vi "createInclinationFrame.vi"(8 "error in (no error)":errorcluster, 9 "TriggerIRQ":bool, 10 "WaitForTrigger":bool, 11 "MIILC in":refnum<class "MIILC.lvclass">) -> (0 "error out":errorcluster, 2 "TxFrame":T1 {"Data" format="%02x"}, 3 "MIILC out":refnum<class "MIILC.lvclass">)   [LabVIEW 2016, in "RTMIILC.lvlib" / "MIILC.lvclass"]
uses:
  MIILC.lvclass
  D:/Code/Common_RT_ILC/ILC/ILC.lvclass
  Common_RT_Modbus/DataTypes/TxFrame.ctl
  Common_RT_Modbus/DynamicFrameBuilder/DynamicFrameBuilder.lvclass
  MIILC.lvclass/MIILC.ctl
  Common_RT_ILC/ILC/ILC.lvclass/ILC.ctl
  Common_RT_ILC/ILC/ILC.lvclass
  Common_RT_Modbus/RTModbus.lvlib
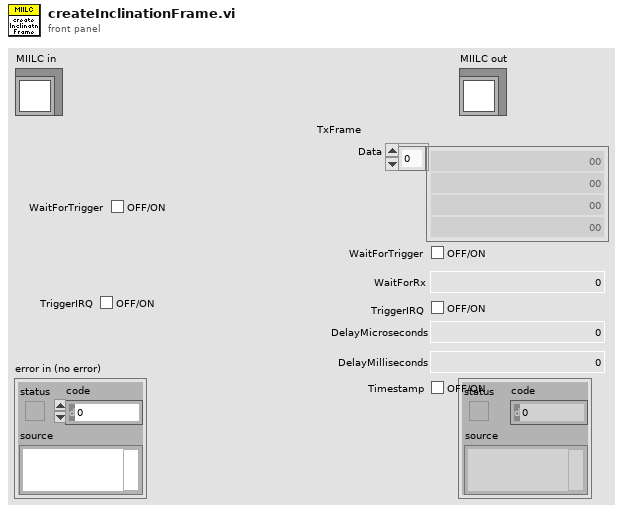
[diagram p1: front panel]
types:
  T1 = typedef "RTModbus.lvlib/TxFrame.ctl" = cluster{"Data":u8[], "WaitForTrigger":bool, "WaitForRx":u16, "TriggerIRQ":bool, "DelayMicroseconds":u16, "DelayMilliseconds":u16, "Timestamp":bool}
  T2 = typedef "RTILC.lvlib/ILCData.ctl" = cluster{"Constants":T3, "Command":T4, "Telemetry":T6, "Responses":T7, "Timings":T9}
  T3 = typedef "RTILC.lvlib/ILCConstants.ctl" = cluster{"Subnet":u8, "Address":u8}
  T4 = typedef "RTILC.lvlib/ILCCommand.ctl" = cluster{"ILCMode":u16, "TemporaryAddress":u8, "ADCScanRate":T5, "ADCChannel":u8, "ADCOffset":sgl, "ADCSensitivity":sgl}
  T5 = typedef "RTILC.lvlib/ILCScanRates.ctl" = u8
  T6 = typedef "RTILC.lvlib/ILCTelemetry.ctl" = cluster{"UniqueID":u64, "FirmwareType":u8, "NetworkNodeType":u8, "ILCOption":u8, "NetworkNodeOption":u8, "MajorRevision":u8, "MinorRevision":u8, "FirmwareName":string, "ILCMode":u16, "MajorFault":bool, "MinorFault":bool, "FaultOverride":bool, "UniqueIDCRCMismatch":bool, "AppTypeNodeTypeMismatch":bool, "AppMissing":bool, "AppCRCMismatch":bool, "TEDSNotFound":bool, "TEDS1Mismatch":bool, "TEDS2Mismatch":bool, "WatchdogResetDetected":bool, "BrownoutDetected":bool, "EventTrapResetDetected":bool, "TemporaryAddress":u8, "ADCScanRate":T5, "DAC1":u16, "DAC2":u16, "DAC3":u16, "DAC4":u16, "MainADCCalibrationK":sgl[], "MainSensorOffset":sgl[], "MainSensorSensitivity":sgl[], "BackupADCCalibrationK":sgl[], "BackupSensorOffset":sgl[], "BackupSensorSensitivity":sgl[]}
  T7 = typedef "RTILC.lvlib/ILCResponses.ctl" = cluster{"ReportServerID":T8, "ReportServerStatus":T8, "ILCMode":T8, "SetTemporaryAddress":T8, "Reset":T8, "ADCScanRate":T8, "ADCOffsetSensitivity":T8, "ReadDAC":T8, "ReadCalibration":T8}
  T8 = typedef "RTModbus.lvlib/ExceptionCodes.ctl" = u16
  T9 = typedef "RTILC.lvlib/ILCTimings.ctl" = cluster{"ADCOffsetSensitivity":u32, "ADCScanRate":u32, "ILCMode":u32, "ReadCalibration":u32, "ReportServerID":u32, "ReportServerStatus":u32, "Reset":u32, "SetTemporaryAddress":u32}
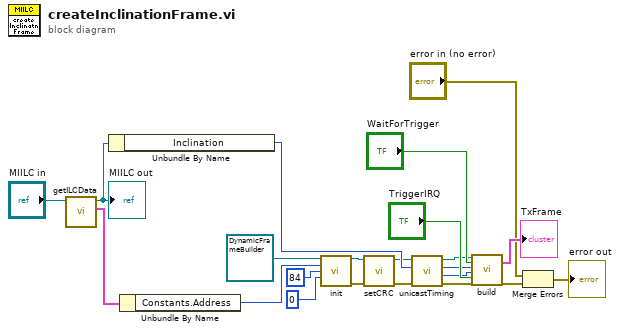
[diagram p0: block diagram]
diagram:
  n1 = call "getILCData.vi"("ILC in"="MIILC in") -> ("ILCData"=w22:T2, "ILC out"=w8:refnum<class "MIILC.lvclass">)  [unwired: 9 in]
  "MIILC out" <- w8
  n2 = Unbundle By Name(w8) -> ("Inclination"=w7:u32)
  n3 = Unbundle By Name(w22) -> ("Constants.Address"=w20:u8)
  n4 = call "init.vi"("DynamicFrameBuilder in"=refnum<class "DynamicFrameBuilder.lvclass"> refnum ("RTModbus.lvlib:DynamicFrameBuilder.lvclass"), "Address"=w20, "Function"=u8 84, "DataSize"=0) -> ("DynamicFrameBuilder out"=w17:refnum<class "DynamicFrameBuilder.lvclass">, "error out"=w14:errorcluster)  [unwired: 10 in]
  n5 = call "setCRC.vi"("error in (no error)"=w14, "DynamicFrameBuilder in"=w17) -> ("error out"=w1:errorcluster, "DynamicFrameBuilder out"=w6:refnum<class "DynamicFrameBuilder.lvclass">)  [unwired: 8 in]
  n6 = call "unicastTiming.vi"("error in (no error)"=w1, "Latency in"=w7, "DynamicFrameBuilder in"=w6) -> ("error out"=w2:errorcluster, "WaitForRxTimeout"=w3:u16, "Latency out"=w4:u32, "DynamicFrameBuilder out"=w5:refnum<class "DynamicFrameBuilder.lvclass">)  [unwired: 5 in]
  n7 = call "build.vi"("DynamicFrameBuilder in"=w5, "WaitForTrigger"="WaitForTrigger", "Latency"=w4, "WaitForRxTimeout"=w3, "TriggerIRQ"="TriggerIRQ", "error in (no error)"=w2) -> ("TxFrame"=→"TxFrame":T1, "error out"=w12:errorcluster)  [unwired: 11 in, 1 out]
  n8 = Merge Errors("error in (no error)", w12) -> (→"error out":errorcluster)
